vi "Player Info.vi"(11 "Wanderer in":refnum<class "Wanderer.lvclass">) -> (1 "Victory Speech":string, 2 "Name":string, 3 "Wanderer out":refnum<class "Wanderer.lvclass">)   [LabVIEW 2015, in "Wanderer.lvclass"]
uses:
  Wanderer.lvclass
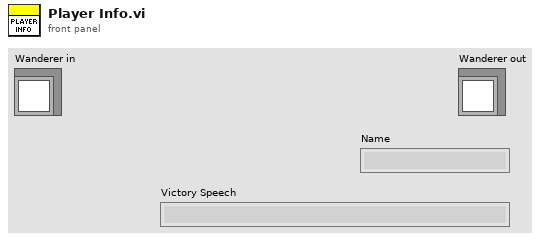
[diagram p1: front panel]
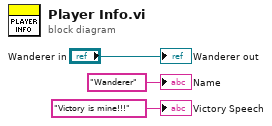
[diagram p0: block diagram]
diagram:
  "Wanderer out" <- "Wanderer in"
  "Name" <- "Wanderer" ("Name")
  "Victory Speech" <- "Victory is mine!!!" ("Victory Speech")
